vi "Highlight File Row.vi"(8 "error in":errorcluster, 9 "Status":string, 10 "Current Row":i32, 11 "Peer Review":refnum<class "Peer Review.lvclass">) -> (0 "error out":errorcluster)   [LabVIEW 2020, in "Peer Review.lvclass"]
uses:
  Peer Review.lvclass
  <vilib>/Utility/miscctls.llb/LVRowAndColumnUnsignedTypeDef.ctl
  Peer Review.lvclass/Peer Review.ctl
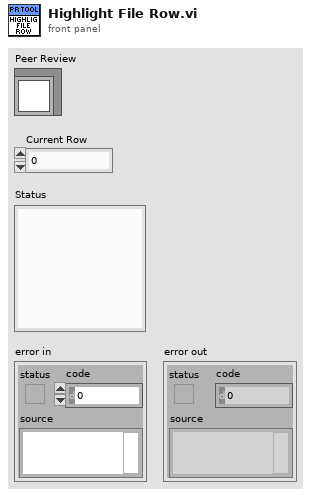
[diagram p1: front panel]
types:
  T1 = typedef "LVRowAndColumnUnsignedTypeDef.ctl" = cluster{"Row":u32, "Column":u32}
  T2 = typedef "Peer Review.lvclass/Compare Info.ctl" = cluster{"File ID":i32, "Commit ID":i32, "Reviewed Hash":string, "Relative Path":string, "File Path":path, "File Checksum":string, "State":T3, "FP Changes":i32, "BD Changes":i32, "Attribute Changes":i32, "Reentrancy Changes":string, "Cyclomatic Complexity":i32, "Node Count":i32, "Version Number":u32, "LabVIEW Version":string, "FP Bounds Error":dbl, "BD Bounds Error":dbl, "Analysis Passes":i32, "Analysis Fails":i32, "Description":string, "Master Path":path, "Master Checksum":string, "VI Type":T4, "LabVIEW File?":bool, "Review Complete?":bool, "File Ref":refnum<vi>}
  T3 = typedef "Peer Review.lvclass/File State.ctl" = enum16{"Interrogation Needed", "Modified", "Deleted", "Added", "Matches Previous", "No Changes", "Moved"}
  T4 = typedef "Peer Review.lvclass/VI Type.ctl" = enum32{"invalid VI type", "Standard VI", "Control VI", "Global VI", "Polymorphic VI", "Configuration VI", "SubSystem", "Facade VI", "Method VI", "Statechart Diagram VI"}
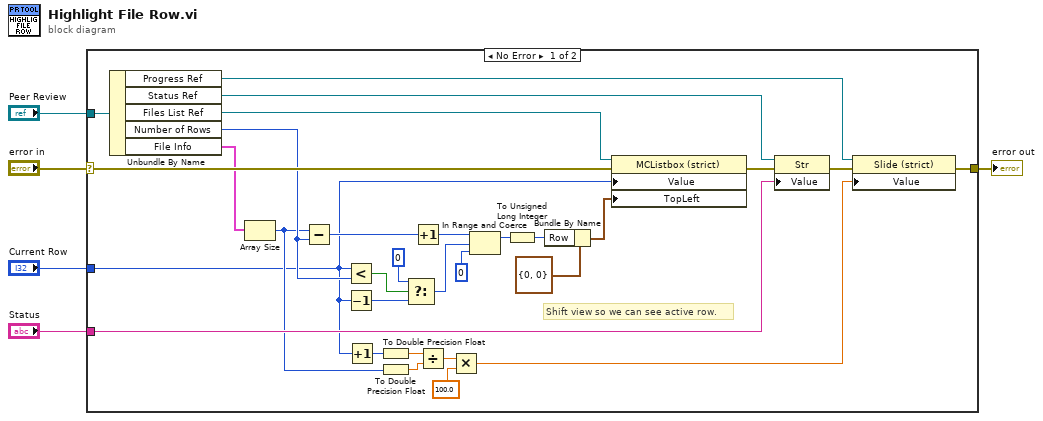
[diagram p0: block diagram]
diagram:
  n1 = case shown="No Error" "error in" {
    selector: "error in" -> [w25 w36]
    tunnel: [w9 w36] -> w4
    tunnel: "Peer Review" -> [w21 _]
    tunnel: "Current Row" -> [w16 _]
    tunnel: "Status" -> [w18 _]
    frame No Error {
      # "Shift view so we can see active row."
      n2 = Unbundle By Name(w21) -> ("Progress Ref"=w6:refnum<vi>, "Status Ref"=w7:refnum<vi>, "Files List Ref"=w23:refnum<vi>, "Number of Rows"=w24:i32, "File Info"=w20:T2[])
      n3 = Array Size(array=w20) -> (size(s)=w17:i32)
      n4 = Subtract(x=w17, y=w24) -> (x-y=w34:i32)
      n5 = Less?(x=w16, y=w24) -> (x < y?=w32:bool)
      n6 = Decrement(x=w16) -> (x-1=w31:i32)
      n7 = Increment(x=w16) -> (x+1=w13:i32)
      n8 = To Double Precision Float(number=w13) -> (double precision float=w14:dbl)
      n9 = To Double Precision Float(number=w17) -> (double precision float=w15:dbl)
      n10 = Select(t=0 ("lower limit"), s=w32, f=w31) -> (s? t:f=w33:i32)
      n11 = Increment(x=w34) -> (x+1=w35:i32)
      n12 = Divide(x=w14, y=w15) -> (x/y=w12:dbl)
      n13 = Multiply(x=w12, y=100.0) -> (x*y=w8:dbl)
      n14 = In Range and Coerce(upper limit=w35, x=w33, lower limit=0) -> (coerced(x)=w26:i32)  [unwired: 1 out]
      n15 = To Unsigned Long Integer(number=w26) -> (unsigned 32bit integer=w22:u32)
      n16 = Bundle By Name(cluster=T1 {"Row"=0, "Column"=0} ("Top Left Visible Cell"), "Row"=w22) -> (w30:T1)
      n17 = property class="MCListbox (strict)"(reference=w23, error in=w25, "Value"=w16, "TopLeft"=w30) -> (error out=w19:errorcluster)  [unwired: 1 out]
      n18 = property class="Str"(reference=w7, error in=w19, "Value"=w18) -> (error out=w10:errorcluster)  [unwired: 1 out]
      n19 = property class="Slide (strict)"(reference=w6, error in=w10, "Value"=w8) -> (error out=w9:errorcluster)  [unwired: 1 out]
    }
    frame Error {
    }
  }
  "error out" <- w4
